vi "SetTCP-NoDelay.vi"(0 "reference in":refnum<class "VdTcpIP.lvclass">, 1 "Connection":refnum<k5>, 2 "TCP_NODELAY (true)":bool=TRUE, 5 "error in (no error)":errorcluster) -> (14 "reference out":refnum<class "VdTcpIP.lvclass">, 19 "error out":errorcluster)   [LabVIEW 2020]
uses:
  <instrlib>/_InstrumentDrivers/VdCommunication/VdTcpIP_class/VdTcpIP.lvclass
  Windows/System32/wsock32.dll
panel:
  # "This is not a member of the class\nSo it's not dragged into all applications.\nProblem for Win XP"
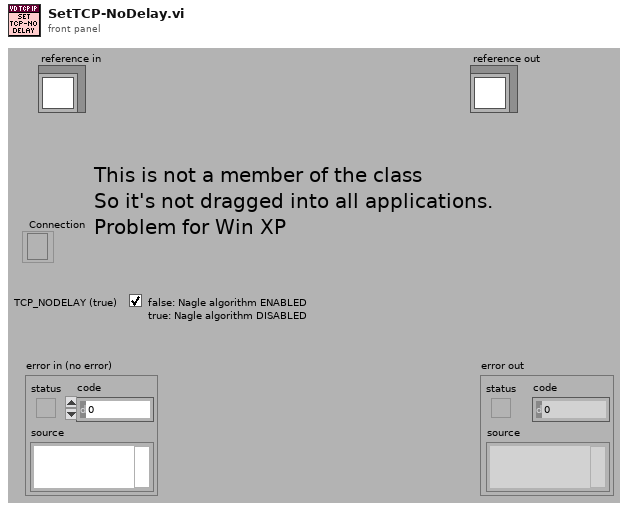
[diagram p1: front panel]
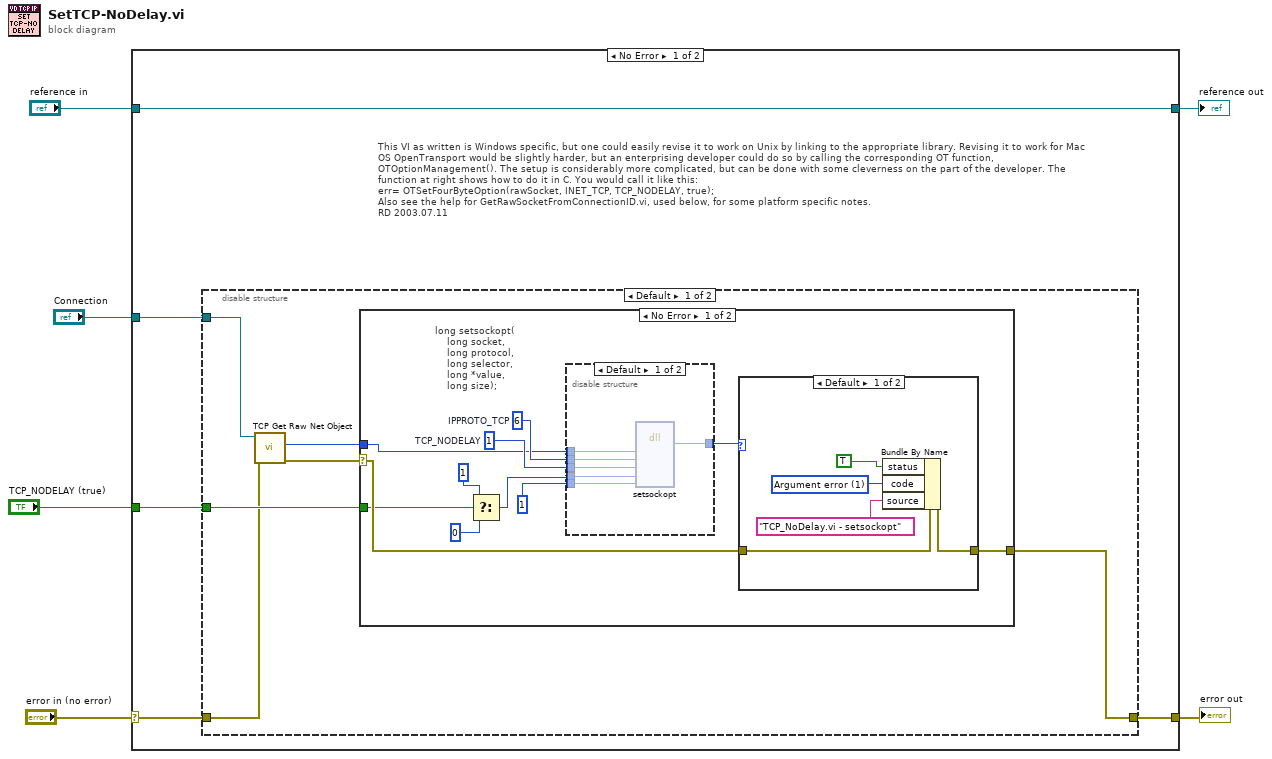
[diagram p0: block diagram]
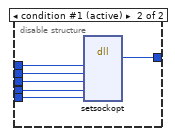
[diagram p2: hidden frame]
diagram:
  n1 = case shown="No Error" "error in (no error)" {
    selector: "error in (no error)" -> [w7 w50]
    tunnel: [w11 w50] -> w5
    tunnel: [w9 w49] -> w3
    tunnel: "reference in" -> [w9 w49]
    tunnel: "TCP_NODELAY (true)" -> [w10 _]
    tunnel: "Connection" -> [w8 _]
    frame No Error {
      # "This VI as written is Windows specific, but one could easily revise it to work on Unix by linking to the appropriate library. Revising it to work for Mac OS OpenTransport would be slightly harder, but an enterprising developer could do so by calling the corresponding OT function, OTOptionManagement(). The setup is considerably more complicated, but can be done with some cleverness on the part of the developer. The function at right shows how to do it in C. You would call it like this:\nerr= OTSetFourByteOption(rawSocket, INET_TCP, TCP_NODELAY, true);\nAlso see the help for GetRawSocketFromConnectionID.vi, used below, for some platform specific notes.\nRD 2003.07.11"
      n2 = disable-structure shown="Default" {
        disable-tunnel: [w15 w48] -> w11
        disable-tunnel: w10 -> [w14 _]
        disable-tunnel: w8 -> [w13 _]
        disable-tunnel: w7 -> [w12 w48]
        frame condition #0 (active) {
          n3 = call <vilib>:"TCP Get Raw Net Object.vi"("error in (no error)"=w12, "connection ID"=w13) -> ("error out"=w17:errorcluster, "raw net object"=w16:u64)  [unwired: 7 in, 1 out]
          n4 = case shown="No Error" w17 {
            selector: w17 -> [w19 w47]
            tunnel: [w21 w47] -> w15
            tunnel: w16 -> [w20 _]
            tunnel: w14 -> [w18 _]
            frame No Error {
              w27 = 1  # TCP_NODELAY
              w28 = 6  # IPPROTO_TCP
              # "long setsockopt(\n    long socket,\n    long protocol,\n    long selector,\n    long *value,\n    long size);"
              n5 = Select(t=u8 1, s=w18, f=u8 0) -> (s? t:f=w24:u8)
              n6 = disable-structure shown="Default" {
                disable-tunnel: w28 -> [w34 w40]
                disable-tunnel: w27 -> [w33 w39]
                disable-tunnel: w24 -> [w32 w38]
                disable-tunnel: 1 ("size") -> [w31 w37]
                disable-tunnel: [w30 w36] -> w22
                disable-tunnel: w20 -> [w29 w35]
                frame condition #0 {
                  n7 = dll-call lib="C:/Windows/System32/wsock32.dll" fn="setsockopt" ("Call Library Function")("socket"=w29, "protocol"=w34, "selector"=w33, "value"=w32, "size"=w31) -> ("return type"=w30:i32)  [unwired: 8 in, 2 out]
                }
                frame condition #1 (active) {
                  n8 = dll-call lib="C:/Windows/System32/wsock32.dll" fn="setsockopt" ("Call Library Function")("socket"=w35, "protocol"=w40, "selector"=w39, "value"=w38, "size"=w37) -> ("return type"=w36:i32)  [unwired: 8 in, 2 out]
                }
              }
              n9 = case shown="Default" w22 {
                tunnel: [w45 w46] -> w21
                tunnel: w19 -> [w41 w46]
                frame Default {
                  w44 = 1 items=["No error", "Argument error", "Memory is full", "Out of zone", "End of file", "File already open", "Generic file I/O error", "File not found", "File permission error", "Disk is full", "Duplicate path", "Too many files open", "System feature not enabled", "Resource file not found", "Cannot add resource", "Resource not found", "Image not found", "Image memory error", "Pen does not exist", "Config type invalid", "Config token not found", "Config parse error", "Config memory error", "Bad external code format", "Bad external code offset", "External code not present", "Null window", "Destroy window error", "Null menu", "Print aborted", "Bad print record", "Print driver error", "Windows error during printing", "Memory error during printing", "Print dialog error", "Generic print error", "Invalid device refnum", "Device not found", "Device parameter error", "Device unit error", "Cannot open device", "Device call aborted", "Generic error", "Cancelled by user", "Object ID too low", "Object ID too high", "Object not in heap", "Unknown heap", "Unknown object (invalid DefProc)", "Unknown object (DefProc not in table)", "Message out of range", "Invalid (null) method", "Unknown message", "Manager call not supported", "Bad address", "Network operation in progress", "Network operation timed out", "Connection is busy", "Network attribute not supported", "Network error", "Address in use", "System out of memory", "Connection aborted", "Connection refused", "Not connected", "Already connected", "Connection closed", "Initialization error (interapplication manager)", "Bad occurrence", "Wait on unbound occurrence handler", "Occurrence queue overflow", "Datalog type conflict", "Unused", "Unrecognized type (interapplication manager)", "Memory corrupt", "Failed to make temporary DLL", "Old CIN version", "Drag socket not found", "Failed to load drop-object", "Failed to register OLE object", "Failed to release OLE object", "Format specifier type mismatch", "Unknown format specifier", "Too few format specifiers", "Too many format specifiers", "Scan failed", "Newer CIN version", "Error converting to variant", "Runtime menu error", "Password tampered", "Variant attribute not found", "Incompatible variant data type", "Event data is not available", "Event Store is not present", "Occurrence is not found", "Event Queue is not created", "Event info is not available", "Refnum passed is NULL", "Error retrieving Class GUID", "Error retrieving CoClass GUID", "Error retrieving TypeLib GUID.", "Bad built application magic bytes.", "Specific driver is different from the specific driver associated with the Logical Name.", "There is no session opened to the class driver.", "Max Error", "MAX - Error with config objects", "MAX - Error loading configuration", "MAX - Group not supported"]
                  n10 = Bundle By Name(cluster=w41, "status"=TRUE, "code"=w44, "source"="TCP_NoDelay.vi - setsockopt") -> (w45:errorcluster)
                }
                frame 0 {
                }
              }
            }
            frame Error {
            }
          }
        }
        frame condition #1 {
        }
      }
    }
    frame Error {
    }
  }
  "error out" <- w5
  "reference out" <- w3
